vi "nominal ingest video.vi"(6 "out_job":i32, 7 "start_ms":dbl, 8 "error in (no error)":errorcluster, 9 "video_rid":string, 10 "file_path":string, 11 "client":i32) -> (0 "error out":errorcluster, 3 "function return":i32, 4 "out_job out":i32)   [LabVIEW 2020, in "client.lvlib"]
doc: "int32_t nominal_ingest_video(int32_t client,\n const char *file_path,\n const char *video_rid,\n double start_ms,\n int32_t *out_job);"
uses:
  client.lvlib
  bin/nominalClient_64.dll
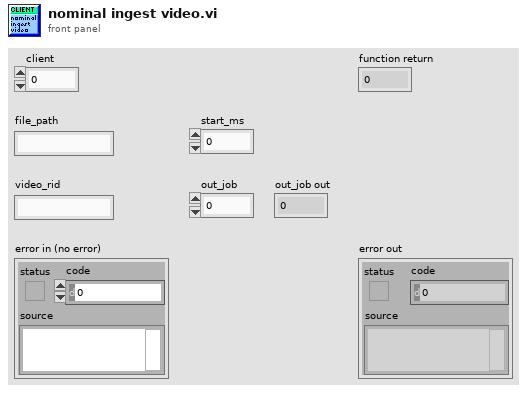
[diagram p1: front panel]
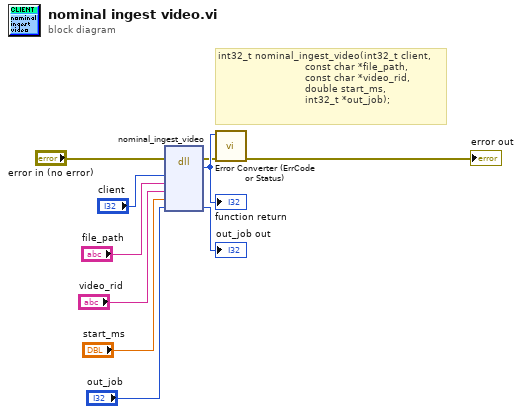
[diagram p0: block diagram]
diagram:
  # "int32_t nominal_ingest_video(int32_t client,\n                             const char *file_path,\n                             const char *video_rid,\n                             double start_ms,\n                             int32_t *out_job);"
  n1 = dll-call lib="C:/code/labview-client-rs/lv_src/bin/nominalClient_*.*" fn="nominal_ingest_video"(error in="error in (no error)", "client"="client", "file_path"="file_path", "video_rid"="video_rid", "start_ms"="start_ms", "out_job"="out_job") -> (error out=w2:errorcluster, w10:i32, "out_job"=→"out_job out":i32)  [unwired: 6 in, 1 out]
  "function return" <- w10
  n2 = call "Error Converter (ErrCode or Status).vi"("error in (no error)"=w2, "error code"=w10) -> ("error out"=→"error out":errorcluster)  [unwired: 9 in]
